vi "Stop All.vi"(8 "error in (no error)":errorcluster, 11 "VacuumLines in":refnum<class "VacuumLines.lvclass">) -> (0 "error out":errorcluster, 3 "VacuumLines out":refnum<class "VacuumLines.lvclass">)   [LabVIEW 2016, in "Hardware.lvlib" / "VacuumLine.lvlib" / "VacuumLines.lvclass"]
uses:
  <userlib>/Common Components/Hardware/Abstract System/VacuumLine/VacuumLines/VacuumLines.lvclass
  <userlib>/Common Components/Hardware/Abstract System/VacuumLine/VacuumLines/VacuumLines.lvclass/VacuumLines.ctl
  <userlib>/Common Components/Hardware/Abstract System/VacuumLine/VacuumLine/VacuumLine.lvclass
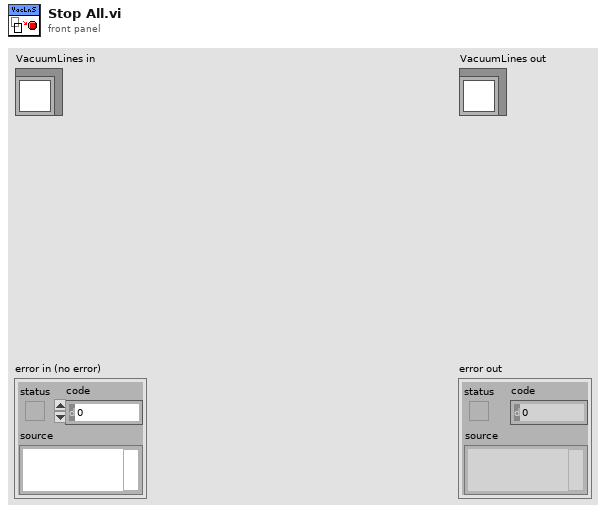
[diagram p1: front panel]
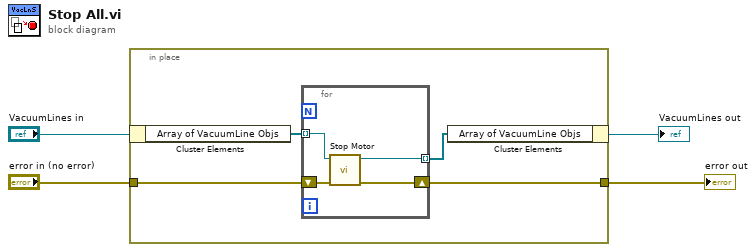
[diagram p0: block diagram]
diagram:
  n1 = in-place {
    in-place-border: "error in (no error)" -> [w7]
    in-place-border: [w5] -> w1
    n2 = in-place-cluster #1("VacuumLines in") -> ("Array of VacuumLine Objs"=w8:refnum<class "VacuumLine.lvclass">[])
    n3 = for {
      tunnel: w8 -> [w10] mode=indexing
      tunnel: [w9] -> w6 mode=indexing
      shift-right: [w11] -> w5
      shift-left: w7 -> [w12]
      n4 = call <userlib>:"Stop Motor.vi"("error in (no error)"=w12, "VacuumLine in"=w10) -> ("error out"=w11:errorcluster, "VacuumLine out"=w9:refnum<class "VacuumLine.lvclass">)  [unwired: 8 in]
    }
    n5 = in-place-cluster #1("Array of VacuumLine Objs"=w6) -> (→"VacuumLines out":refnum<class "VacuumLines.lvclass">)
  }
  "error out" <- w1
